vi "Temperature Conversion.vi"() -> ()   [LabVIEW 2022 SP3]
panel:
  in  "stop":bool
  out "Celcius":dbl
  out "Celcius Chart":dbl(graph)
  in  "Fahrenheit":dbl
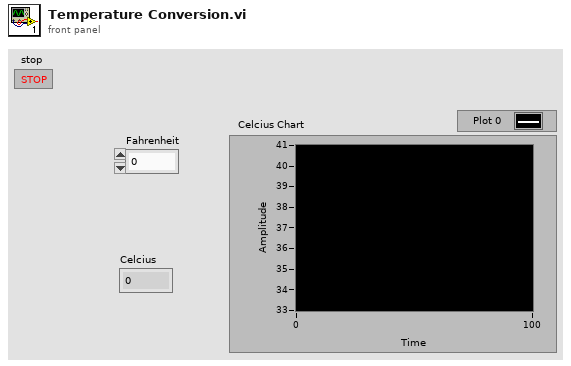
[diagram p1: front panel]
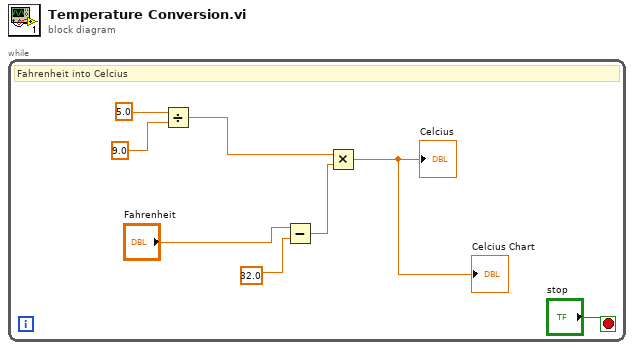
[diagram p0: block diagram]
diagram:
  n1 = while {
    stop <- "stop" stop-if-true
    # "Fahrenheit into Celcius"
    n2 = Divide(x=5.0 ("x/y"), y=9.0) -> (x/y=w4:dbl)
    n3 = Subtract(x="Fahrenheit", y=32.0 ("x-y")) -> (x-y=w3:dbl)
    n4 = Multiply(x=w4, y=w3) -> (x*y=→"Celcius Chart" →"Celcius":dbl)
  }
